vi "Teleop.vi"(10 "Match Info":T1={"Autonomous Elapsed Seconds"=0.0, "TeleOp Elapsed Seconds"=0.0, "Disabled Elapsed Seconds"=0.0, "Visited Autonomous"=FALSE, "Visited TeleOp"=FALSE, "Visited Disabled"=FALSE, "Autonomous Settings"={"Autonomous Style"=enum."Independent", "VI Refnum"=refnum}}, 11 "Call Context":T2) -> ()   [LabVIEW 2019]
doc: "This VI is called for each enabled TeleOp packet received from the DS. It is typically used to read from joysticks and other inputs and update I/O or setpoints for timed control loops. It should complete and return within 20 milliseconds or risk missing DS packets."
uses:
  <vilib>/Rock Robotics/WPI/DriverStation/WPI_DriverStationDerivedRobotMode.ctl
  <vilib>/Rock Robotics/WPI/DriverStation/WPI_DriverStationMatch Info.ctl
  Framework/Robot Global Data.vi
  <vilib>/Rock Robotics/Network Tables/NT Write Boolean.vi
  <vilib>/Rock Robotics/Network Tables/NT Write Number.vi
  <vilib>/Rock Robotics/Network Tables/NT Write Numeric Array.vi
  <vilib>/Rock Robotics/Network Tables/NT Write Boolean Array.vi
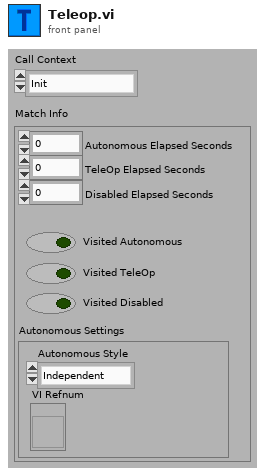
[diagram p1: front panel]
types:
  T1 = typedef "WPI_DriverStationMatch Info.ctl" = cluster{"Autonomous Elapsed Seconds":dbl, "TeleOp Elapsed Seconds":dbl, "Disabled Elapsed Seconds":dbl, "Visited Autonomous":bool, "Visited TeleOp":bool, "Visited Disabled":bool, "Autonomous Settings":cluster{"Autonomous Style":enum16{"Iterative", "Independent"}, "VI Refnum":refnum<vi>}}
  T2 = typedef "WPI_DriverStationDerivedRobotMode.ctl" = enum16{"Init", "Execute", "Stop"}
  T3 = typedef "WPI_JoystickDevRef.ctl" = cluster{"Device":T4}
  T4 = typedef "WPI_JoystickDeviceEnum.ctl" = enum16{"USB 0", "USB 1", "USB 2", "USB 3", "USB 4", "USB 5"}
  T5 = typedef "Command Status Info.ctl" = cluster{"Name":string, "Status":T6, "notifier out":T7}
  T6 = typedef "Completion Status.ctl" = enum16{"Successful", "Aborted", "Incomplete"}
  T7 = typedef "Completion Notifier.ctl" = refnum<notifier>
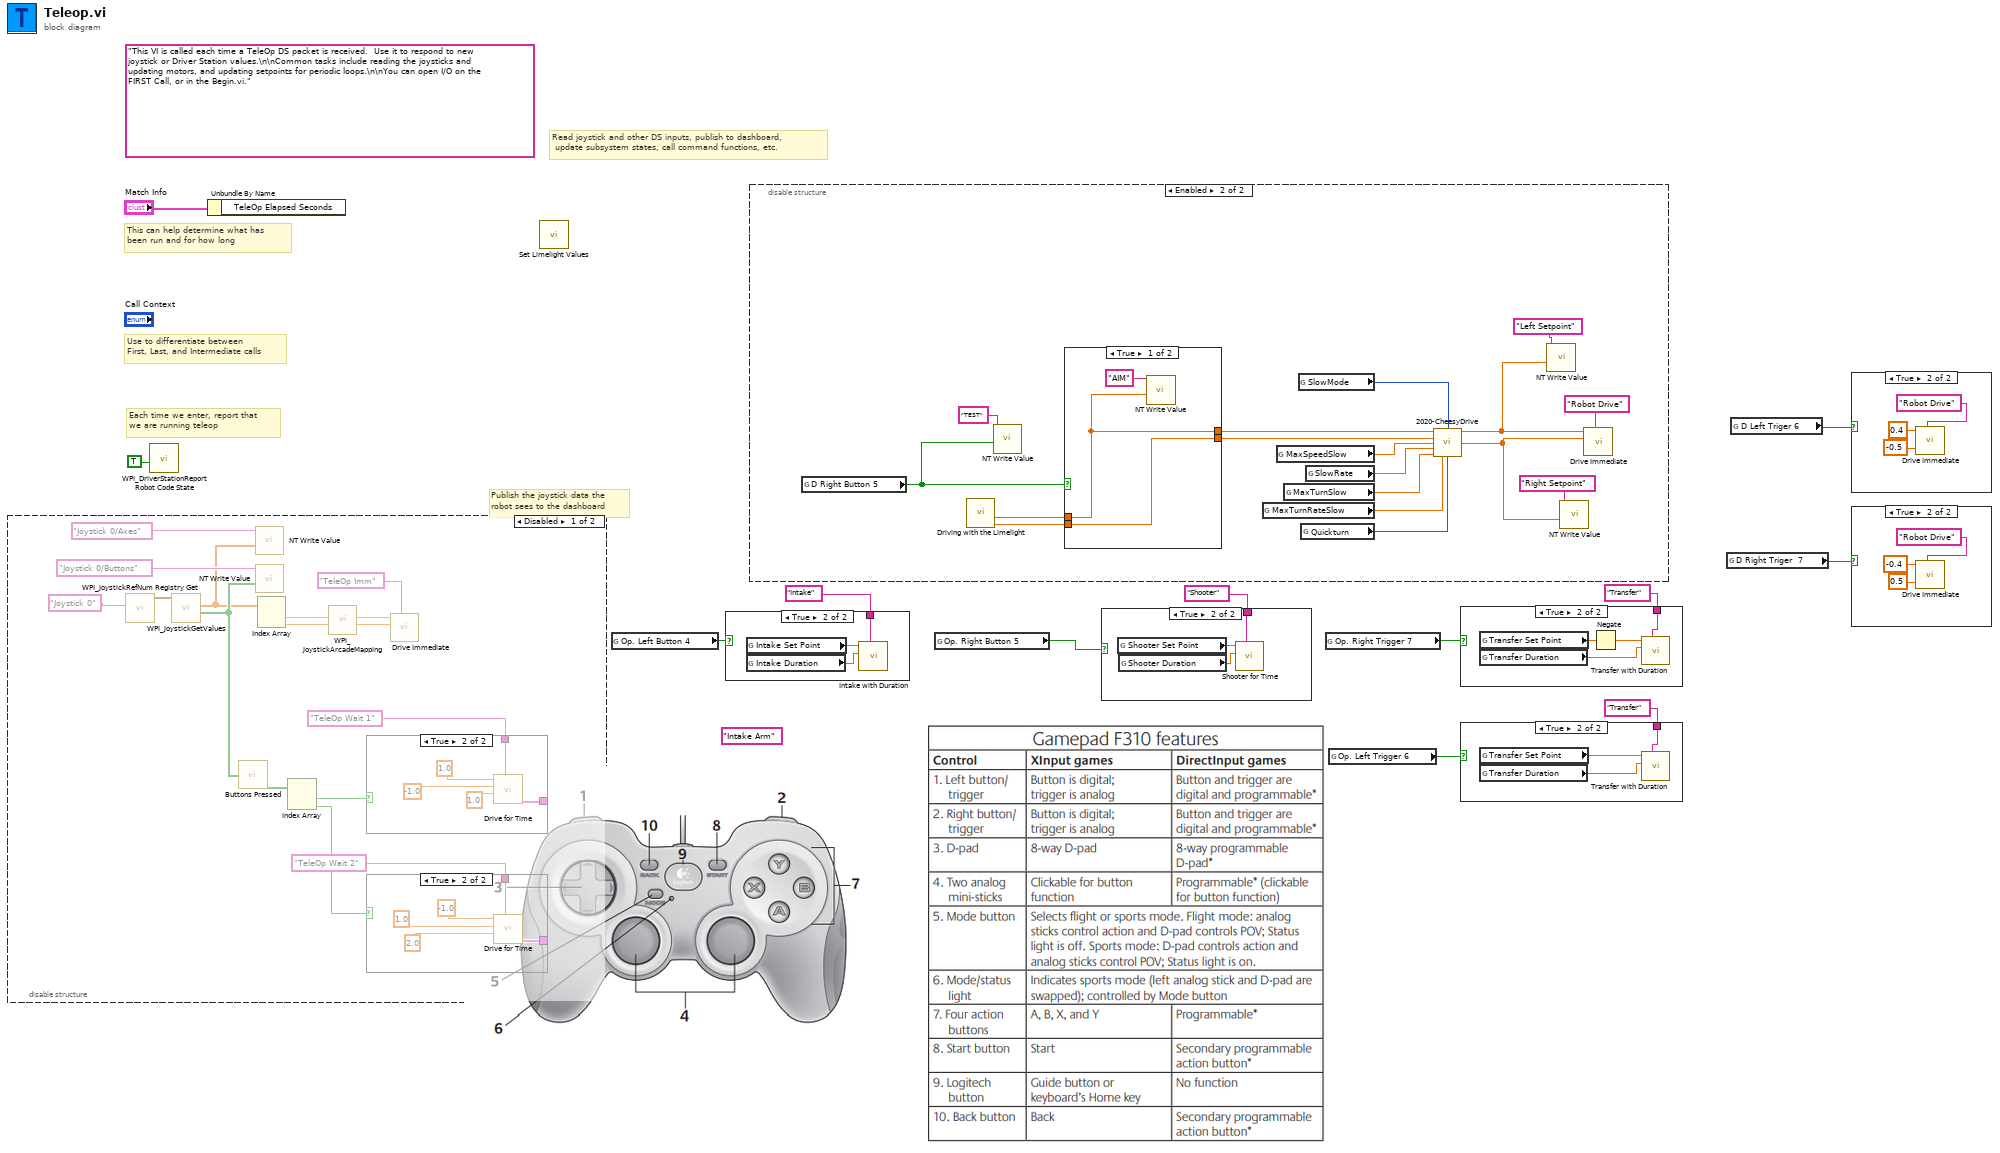
[diagram p0: block diagram]
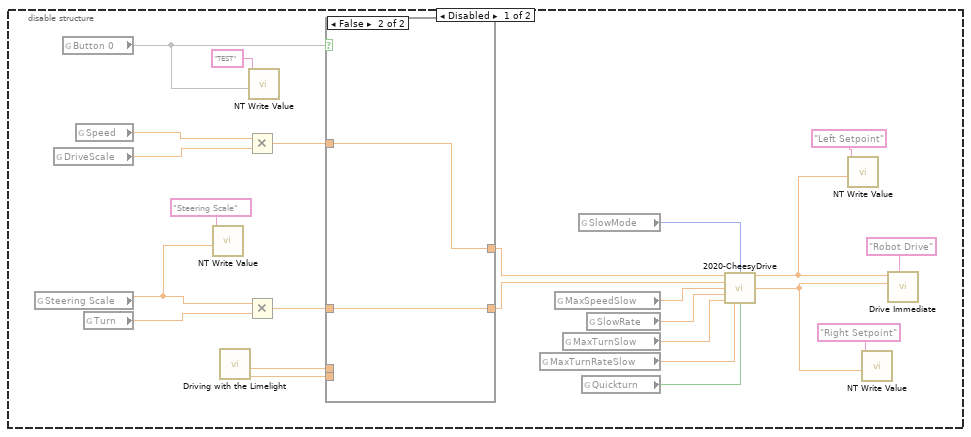
[diagram p8: hidden frame]
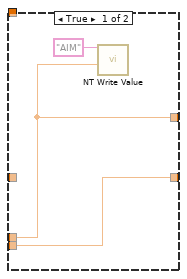
[diagram p9: hidden frame]
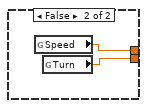
[diagram p10: hidden frame]
diagram:
  (unwired) "Intake Arm" ("refnum name")
  (unwired) "This VI is called each time a TeleOp DS packet is received.  Use it to respond to new joystick or Driver Station values.\n\nCommon tasks include reading the joysticks and updating motors, and updating setpoints for periodic loops.\n\nYou can open I/O on the FIRST Call, or in the Begin.vi."
  # "Publish the joystick data the\nrobot sees to the dashboard"
  # "Read joystick and other DS inputs, publish to dashboard,\n update subsystem states, call command functions, etc."
  # "Each time we enter, report that\nwe are running teleop"
  # "Use to differentiate between\nFirst, Last, and Intermediate calls"
  # "This can help determine what has\nbeen run and for how long"
  n1 = disable-structure shown="Disabled" {
    frame Disabled {
      n2 = call <vilib>:"WPI_JoystickRefNum Registry Get.vi"("refnum name"="Joystick 0") -> ("JoystickDevRef"=w27:T3)  [unwired: 1 in, 9 out]
      n3 = call <vilib>:"WPI_JoystickGetValues.vi"("JoystickDevRef"=w27) -> ("Buttons"=w15:bool[], "Axes"=w14:dbl[])  [unwired: 6 in, 3 out]
      n4 = call "Buttons Pressed.vi"("Button Values"=w15) -> ("Button Presses"=w23:bool[])
      n5 = call-poly <vilib>:"NT Write Value.vi"("Numeric Array"=w14, "Name"="Joystick 0/Axes") -> ()  [unwired: 9 in, 1 out]
      n6 = call-poly <vilib>:"NT Write Value.vi"("Boolean Array"=w15, "Name"="Joystick 0/Buttons") -> ()  [unwired: 9 in, 1 out]
      n7 = Index Array(array=w14) -> (element #1=w18:dbl, element #2=w17:dbl)  [unwired: 2 in]
      n8 = Index Array(array=w23) -> (element #1=w22:bool, element #2=w21:bool)  [unwired: 2 in]
      n9 = call <vilib>:"WPI_JoystickArcadeMapping.vi"("Y axis value"=w17, "X axis value"=w18) -> ("Right Motor Value"=w19:dbl, "Left Motor Value"=w20:dbl)  [unwired: 8 in]
      n10 = case shown="True" w22 {
        tunnel: [_ w37] -> _
        tunnel: "TeleOp Wait 1" ("Description") -> [_ w36]
        frame False {
        }
        frame True {
          n11 = call "Drive for Time.vi"("Description"=w36, "Seconds"=1.0, "Right Speed"=-1.0, "Left Speed"=1.0) -> ("Command Info Out"=w37:T5)  [unwired: 7 in]
        }
      }
      n12 = case shown="True" w21 {
        tunnel: [_ w31] -> _
        tunnel: "TeleOp Wait 2" ("Description") -> [_ w30]
        frame False {
        }
        frame True {
          n13 = call "Drive for Time.vi"("Description"=w30, "Seconds"=2.0, "Right Speed"=1.0, "Left Speed"=-1.0) -> ("Command Info Out"=w31:T5)  [unwired: 7 in]
        }
      }
      n14 = call "Drive Immediate.vi"("Description"="TeleOp Imm", "Right Setpoint"=w19, "Left Setpoint"=w20) -> ()  [unwired: 8 in, 1 out]
    }
    frame Enabled {
    }
  }
  n15 = call <vilib>:"WPI_DriverStationReport Robot Code State.vi"("TeleOp"=TRUE ("Autonomous")) -> ()  [unwired: 10 in, 1 out]
  n16 = Unbundle By Name("Match Info") -> ()  [unwired: 1 out]
  n17 = call "Set Limelight Values.vi"() -> ()  [unwired: 12 in]
  n18 = global read "Robot Global Data.vi" "Op. Left Button 4"() -> (w10:bool)
  n19 = case shown="True" w10 {
    tunnel: "Intake" ("refnum name") -> [_ w41]
    frame False {
    }
    frame True {
      n20 = global read "Robot Global Data.vi" "Intake Set Point"() -> (w40:dbl)
      n21 = global read "Robot Global Data.vi" "Intake Duration"() -> (w39:dbl)
      n22 = call "Intake with Duration.vi"("Description"=w41, "Duration (s)"=w39, "Setpoint"=w40) -> ()  [unwired: 8 in, 1 out]
    }
  }
  n23 = disable-structure shown="Enabled" {
    frame Disabled {
      n24 = global read "Robot Global Data.vi" "Steering Scale"() -> (w43:dbl)
      n25 = global read "Robot Global Data.vi" "DriveScale"() -> (w42:dbl)
      n26 = global read "Robot Global Data.vi" "Button 0"() -> (w52)
      n27 = global read "Robot Global Data.vi" "Speed"() -> (w53:dbl)
      n28 = global read "Robot Global Data.vi" "Turn"() -> (w54:dbl)
      n29 = call-poly <vilib>:"NT Write Value.vi"("Numeric"=w43, "Name"="Steering Scale") -> ()  [unwired: 9 in, 1 out]
      n30 = call "Driving with the Limelight.vi"() -> ("TurnCommand"=w58:dbl, "SpeedCommand"=w57:dbl)  [unwired: 9 in, 1 out]
      n31 = Multiply(x=w53, y=w42) -> (x*y=w63:dbl)
      n32 = Multiply(x=w43, y=w54) -> (x*y=w64:dbl)
      n33 = call-poly <vilib>:"NT Write Value.vi"("Boolean"=w52, "Name"="TEST") -> ()  [unwired: 9 in, 1 out]
      n34 = case shown="False" w52 {
        tunnel: w64 -> [_ w70]
        tunnel: w63 -> [_ w69]
        tunnel: [w67 w69] -> w61
        tunnel: w58 -> [w66 _]
        tunnel: w57 -> [w67 _]
        tunnel: [w66 w70] -> w55
        frame True {
          n35 = call-poly <vilib>:"NT Write Value.vi"("Numeric"=w67, "Name"="AIM") -> ()  [unwired: 9 in, 1 out]
        }
        frame False {
        }
      }
      n36 = global read "Robot Global Data.vi" "MaxTurnRateSlow"() -> (w44:dbl)
      n37 = global read "Robot Global Data.vi" "MaxSpeedSlow"() -> (w47:dbl)
      n38 = global read "Robot Global Data.vi" "MaxTurnSlow"() -> (w45:dbl)
      n39 = global read "Robot Global Data.vi" "SlowMode"() -> (w60:u32)
      n40 = global read "Robot Global Data.vi" "Quickturn"() -> (w56:bool)
      n41 = global read "Robot Global Data.vi" "SlowRate"() -> (w46:dbl)
      n42 = call "2020-CheesyDrive.vi"("Throttle"=w61, "SlowMode"=w60, "Wheel"=w55, "MaxSpeedSlow"=w47, "SlowRate"=w46, "MaxTurnSlow"=w45, "MaxTurnRateSlow"=w44, "Quickturn"=w56) -> ("Left PWM"=w49:dbl, "Right PWM"=w48:dbl)  [unwired: 6 in]
      n43 = call-poly <vilib>:"NT Write Value.vi"("Numeric"=w49, "Name"="Left Setpoint") -> ()  [unwired: 9 in, 1 out]
      n44 = call-poly <vilib>:"NT Write Value.vi"("Numeric"=w48, "Name"="Right Setpoint") -> ()  [unwired: 9 in, 1 out]
      n45 = call "Drive Immediate.vi"("Description"="Robot Drive", "Right Setpoint"=w48, "Left Setpoint"=w49) -> ()  [unwired: 8 in, 1 out]
    }
    frame Enabled {
      n46 = global read "Robot Global Data.vi" "D Right Button 5"() -> (w79:bool)
      n47 = call "Driving with the Limelight.vi"() -> ("TurnCommand"=w83:dbl, "SpeedCommand"=w82:dbl)  [unwired: 9 in, 1 out]
      n48 = call-poly <vilib>:"NT Write Value.vi"("Boolean"=w79, "Name"="TEST") -> ()  [unwired: 9 in, 1 out]
      n49 = case shown="True" w79 {
        tunnel: [w89 w92] -> w86
        tunnel: w83 -> [w88 _]
        tunnel: w82 -> [w89 _]
        tunnel: [w88 w91] -> w80
        frame True {
          n50 = call-poly <vilib>:"NT Write Value.vi"("Numeric"=w89, "Name"="AIM") -> ()  [unwired: 9 in, 1 out]
        }
        frame False {
          n51 = global read "Robot Global Data.vi" "Speed"() -> (w92:dbl)
          n52 = global read "Robot Global Data.vi" "Turn"() -> (w91:dbl)
        }
      }
      n53 = global read "Robot Global Data.vi" "MaxTurnRateSlow"() -> (w71:dbl)
      n54 = global read "Robot Global Data.vi" "MaxSpeedSlow"() -> (w74:dbl)
      n55 = global read "Robot Global Data.vi" "MaxTurnSlow"() -> (w72:dbl)
      n56 = global read "Robot Global Data.vi" "SlowMode"() -> (w85:u32)
      n57 = global read "Robot Global Data.vi" "Quickturn"() -> (w81:bool)
      n58 = global read "Robot Global Data.vi" "SlowRate"() -> (w73:dbl)
      n59 = call "2020-CheesyDrive.vi"("Throttle"=w86, "SlowMode"=w85, "Wheel"=w80, "MaxSpeedSlow"=w74, "SlowRate"=w73, "MaxTurnSlow"=w72, "MaxTurnRateSlow"=w71, "Quickturn"=w81) -> ("Left PWM"=w76:dbl, "Right PWM"=w75:dbl)  [unwired: 6 in]
      n60 = call-poly <vilib>:"NT Write Value.vi"("Numeric"=w76, "Name"="Left Setpoint") -> ()  [unwired: 9 in, 1 out]
      n61 = call-poly <vilib>:"NT Write Value.vi"("Numeric"=w75, "Name"="Right Setpoint") -> ()  [unwired: 9 in, 1 out]
      n62 = call "Drive Immediate.vi"("Description"="Robot Drive", "Right Setpoint"=w75, "Left Setpoint"=w76) -> ()  [unwired: 8 in, 1 out]
    }
  }
  n63 = global read "Robot Global Data.vi" "Op. Right Button 5"() -> (w6:bool)
  n64 = case shown="True" w6 {
    tunnel: "Shooter" ("refnum name") -> [_ w95]
    frame False {
    }
    frame True {
      n65 = global read "Robot Global Data.vi" "Shooter Set Point"() -> (w94:dbl)
      n66 = global read "Robot Global Data.vi" "Shooter Duration"() -> (w93:dbl)
      n67 = call "Shooter for Time.vi"("Description"=w95, "Duration (s)"=w93, "Setpoint"=w94) -> ()  [unwired: 8 in, 1 out]
    }
  }
  n68 = global read "Robot Global Data.vi" "Op. Right Trigger 7"() -> (w5:bool)
  n69 = global read "Robot Global Data.vi" "Op. Left Trigger 6"() -> (w4:bool)
  n70 = case shown="True" w5 {
    tunnel: "Transfer" ("refnum name") -> [_ w99]
    frame False {
    }
    frame True {
      n71 = global read "Robot Global Data.vi" "Transfer Set Point"() -> (w97:dbl)
      n72 = global read "Robot Global Data.vi" "Transfer Duration"() -> (w96:dbl)
      n73 = Negate(x=w97) -> (-x=w98:dbl)
      n74 = call "Transfer with Duration.vi"("Description"=w99, "Duration (s)"=w96, "Setpoint"=w98) -> ()  [unwired: 8 in, 1 out]
    }
  }
  n75 = case shown="True" w4 {
    tunnel: "Transfer" ("refnum name") -> [_ w102]
    frame False {
    }
    frame True {
      n76 = global read "Robot Global Data.vi" "Transfer Set Point"() -> (w101:dbl)
      n77 = global read "Robot Global Data.vi" "Transfer Duration"() -> (w100:dbl)
      n78 = call "Transfer with Duration.vi"("Description"=w102, "Duration (s)"=w100, "Setpoint"=w101) -> ()  [unwired: 8 in, 1 out]
    }
  }
  n79 = global read "Robot Global Data.vi" "D Right Triger  7"() -> (w1:bool)
  n80 = global read "Robot Global Data.vi" "D Left Triger 6"() -> (w2:bool)
  n81 = case shown="True" w2 {
    frame False {
    }
    frame True {
      n82 = call "Drive Immediate.vi"("Description"="Robot Drive", "Right Setpoint"=-0.5, "Left Setpoint"=0.4) -> ()  [unwired: 8 in, 1 out]
    }
  }
  n83 = case shown="True" w1 {
    frame False {
    }
    frame True {
      n84 = call "Drive Immediate.vi"("Description"="Robot Drive", "Right Setpoint"=0.5, "Left Setpoint"=-0.4) -> ()  [unwired: 8 in, 1 out]
    }
  }
